vi "DetermineHeadingRegimeTest.vi"() -> (3 "Were there any errors at all?":bool)   [LabVIEW 2013]
uses:
  Data/TypeDefs/Sailing Regimes.ctl
  Data/TypeDefs/Regime Boundaries.ctl
panel:
  in  "Expected Chosen Regime Outputs":T1[](array[typedef])=[enum."Reach - Port Tack", enum."Upwind - Starboard Tack", enum."Run - Starboard Tack"]
  in  "Robot Heading":dbl[](array[numeric])=[90.0, 5.0, 153.0]
  in  "Trusted Absolute Wind Data":dbl[](array[numeric])=[181.0, 355.0, 1.0]
  out "Actual Chosen Regime Outputs":T1[](array[typedef])
  out "Are chosen distances right?":bool[](array[boolean])=[TRUE, TRUE, TRUE, TRUE, TRUE, TRUE]
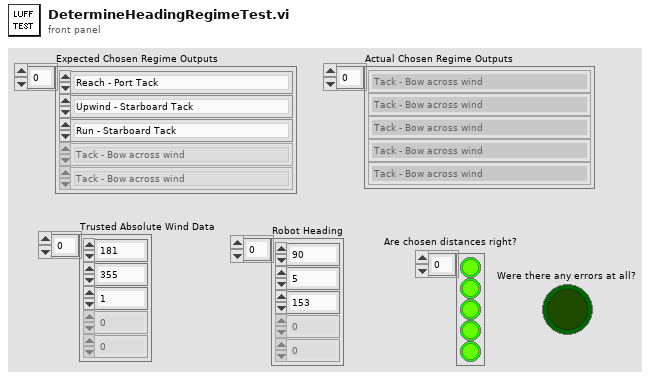
[diagram p1: front panel]
types:
  T1 = typedef "Sailing Regimes.ctl" = enum16{"Tack - Bow across wind", "Upwind - Starboard Tack", "Turn between Upwind/Reach - Starboard Tack", "Reach - Starboard Tack", "Turn between Reach/Run - Starboard Tack", "Run - Starboard Tack", "Jibe - Stern across wind", "Run - Port Tack", "Turn between Reach/Run - Port Tack", "Reach - Port Tack", "Turn between Upwind/Reach - Port Tack", "Upwind - Port Tack"}
  T2 = typedef "Regime Boundaries.ctl" = i32[]
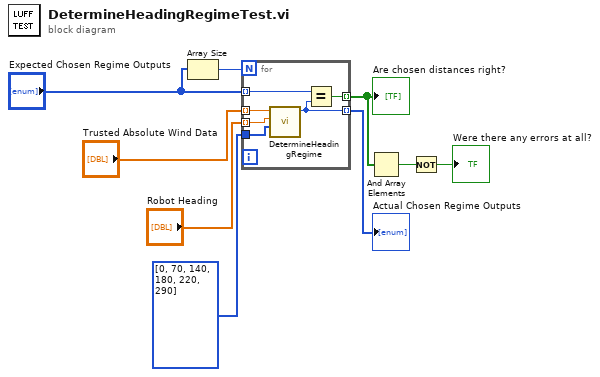
[diagram p0: block diagram]
diagram:
  n1 = Array Size(array="Expected Chosen Regime Outputs") -> (size(s)=w9:i32)
  n2 = for {
    N: w9 -> [_]
    tunnel: [w15] -> w8 mode=indexing
    tunnel: [w11] -> w6 mode=indexing
    tunnel: "Expected Chosen Regime Outputs" -> [w14] mode=indexing
    tunnel: "Trusted Absolute Wind Data" -> [w13] mode=indexing
    tunnel: "Robot Heading" -> [w12] mode=indexing
    tunnel: T2 [0, 70, 140, 180, 220, 290] ("Altered regime boundaries") -> [w10]
    n3 = call "DetermineHeadingRegime.vi"("Altered regime boundaries"=w10, "Robot Heading (deg)"=w12, "Trusted Absolute Wind Data (deg)"=w13) -> ("Sailing Regime"=w11:T1)  [unwired: 8 in]
    n4 = Equal?(x=w14, y=w11) -> (x = y?=w15:bool)
  }
  "Are chosen distances right?" <- w8
  "Actual Chosen Regime Outputs" <- w6
  n5 = And Array Elements(Boolean array=w8) -> (logical AND=w5:bool)
  n6 = Not(x=w5) -> (.not. x?=→"Were there any errors at all?":bool)
